vi "MEMR-Flush IPC.vi"(7 "IPC":T1) -> (8 "IPC thru":T1, 15 "error out":errorcluster)   [LabVIEW 2020]
uses:
  Typedefs/MEMR-IPC.ctl
  Typedefs/MEMR-Params.ctl
  Typedefs/MEMR-Probe.ctl
  Typedefs/MEMR-Elicitor.ctl
  Human Studies/SFM Frontend/LV Source/Typedefs/HSTS-Transducer.ctl
  Typedefs/MEMR-Sequence.ctl
  Typedefs/MEMR-Analysis.ctl
  Typedefs/MEMR-Timing.ctl
  CFTS Main Panel SubVIs/CFTS-Experiment State.ctl
  Typedefs/MEMR-Sequence Step.ctl
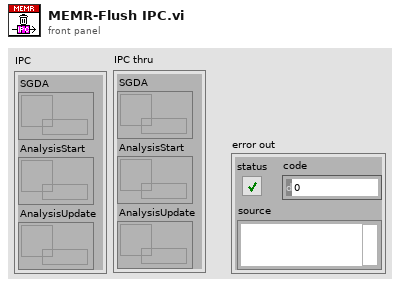
[diagram p1: front panel]
types:
  T1 = typedef "MEMR-IPC.ctl" = cluster{"SGDA":refnum<queue>, "AnalysisStart":refnum<queue>, "AnalysisUpdate":refnum<queue>}
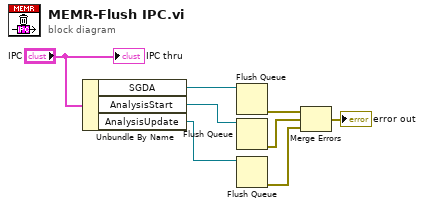
[diagram p0: block diagram]
diagram:
  n1 = Unbundle By Name("IPC") -> ("SGDA"=w7:refnum<queue>, "AnalysisStart"=w6:refnum<queue>, "AnalysisUpdate"=w5:refnum<queue>)
  n2 = Flush Queue(queue=w7) -> (error out=w4:errorcluster)  [unwired: 1 in, 2 out]
  n3 = Flush Queue(queue=w6) -> (error out=w3:errorcluster)  [unwired: 1 in, 2 out]
  n4 = Flush Queue(queue=w5) -> (error out=w2:errorcluster)  [unwired: 1 in, 2 out]
  n5 = Merge Errors(w4, w3, w2) -> (→"error out":errorcluster)
  "IPC thru" <- "IPC"
